vi "Host to DMA FIFO test.vi"() -> ()   [LabVIEW 2019]
uses:
  GlobalVars.vi
  <vilib>/FPGAPlugInAG/sbRIO-9606/niLvFpga_Open_sbRIO-9606.vi
  <vilib>/rvi/interface/common/dynamic/niFpgaDynamicAddResources.vi
  <vilib>/FPGAPlugInAG/Dynamic/niLvFpga_Abort_Dynamic.vi
  <vilib>/FPGAPlugInAG/Dynamic/niLvFpga_Reset_Dynamic.vi
  <vilib>/Utility/error.llb/Error Cluster From Error Code.vi
  <vilib>/rvi/errors/niLvFpgaAdjustHostInterfaceError.vi
  <vilib>/FPGAPlugInAG/Dynamic/niLvFpga_Run_Dynamic.vi
  <vilib>/FPGAPlugInAG/Dynamic/niLvFpga_Close_Dynamic.vi
  <vilib>/rvi/interface/nirviOpenFPGA/nirviOpenFPGA.xnode
  FPGA Bitfiles/sbriotest_MainFPGATarget_MainDMAFIFOtest_3lPTgoDMRHg.lvbitx
  Main DMA FIFO test.vi
  FPGA Bitfiles/sbriotest_SecondFPGATarget_AuxDMAFIFOtest_dfB-yokIQYE.lvbitx
  Aux DMA FIFO test.vi
  <vilib>/rvi/interface/nirviMethod/nirviMethod.xnode
  <vilib>/rvi/interface/nirviReadWriteControl/nirviReadWriteControl.xnode
  <vilib>/rvi/interface/nirviCloseFPGA/nirviCloseFPGA.xnode
  NiFpgaLv.dll
  <vilib>/rvi/interface/Simulation/niFpgaSimulationCallBeginRW.vi
  <vilib>/FPGAPlugInAG/Dynamic/niLvFpga_WriteFifo_Dynamic.vi
  <vilib>/rvi/errors/niLvFpgaMergeErrorWithErrorCode.vi
  <vilib>/FPGAPlugInAG/Dynamic/niLvFpga_ReadFifo_Dynamic.vi
panel:
  out "aux xt counter":u32
  out "both pass":bool
  out "GBIP total":i32
  out "xt counter":u32
  out "diff [us]":i32
  out "elapsed aux":u32
  out "GBIP command":string
  out "xt length":u32
  out "xt end":u32
  in  "stop":bool
  out "elapsed":u32
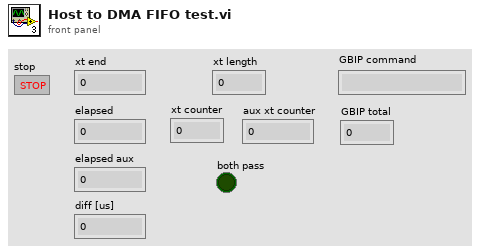
[diagram p1: front panel]
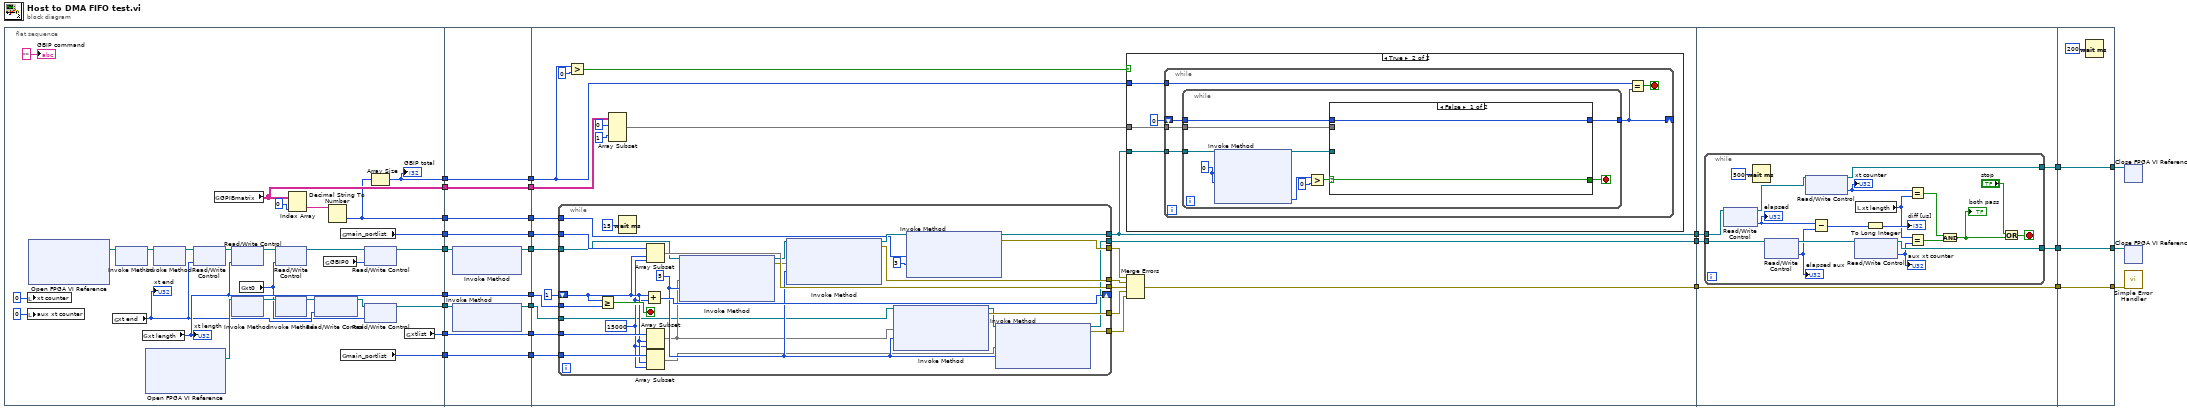
[diagram p0: block diagram]
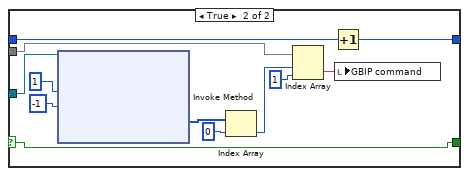
[diagram p3: hidden frame]
diagram:
  n1 = flat-sequence {
    tunnel: [w53] -> w21
    tunnel: [w52] -> w19
    tunnel: [w45] -> w17
    tunnel: [w49] -> w15
    tunnel: [w39] -> w13
    tunnel: [w36] -> w11
    tunnel: [w37] -> w9
    tunnel: [w32] -> w7
    tunnel: [w30] -> w6
    tunnel: w21 -> [w65]
    tunnel: [w65] -> w20
    tunnel: w19 -> [w64]
    tunnel: [w64] -> w18
    tunnel: w17 -> [w63]
    tunnel: [w63] -> w16
    tunnel: w15 -> [w62]
    tunnel: [w62] -> w14
    tunnel: w13 -> [w61]
    tunnel: [w61] -> w12
    tunnel: w11 -> [w60]
    tunnel: [w60] -> w10
    tunnel: w9 -> [w59]
    tunnel: [w59] -> w8
    tunnel: w7 -> [w58]
    tunnel: w6 -> [w57]
    tunnel: [w56] -> w5
    tunnel: [w55] -> w4
    tunnel: w20 -> [w88]
    tunnel: w18 -> [w87]
    tunnel: w16 -> [w84]
    tunnel: w14 -> [w70]
    tunnel: [w85] -> w25
    tunnel: w12 -> [w83]
    tunnel: [w77] -> w24
    tunnel: [w76] -> w22
    tunnel: w10 -> [w68]
    tunnel: w8 -> [w75]
    tunnel: w5 -> [w74]
    tunnel: w4 -> [w73]
    tunnel: w25 -> [w152]
    tunnel: w24 -> [w151]
    tunnel: w22 -> [w150]
    tunnel: [w154] -> w3
    tunnel: [w153] -> w2
    tunnel: [w151] -> w1
    tunnel: [w175] -> w23
    tunnel: [w176] -> w26
    tunnel: [w177] -> w27
    tunnel: w3 -> [w177]
    tunnel: w2 -> [w176]
    tunnel: w1 -> [w175]
    frame #0 {
      n2 = local write "xt counter"(u32 0 ("xt counter")) -> ()
      n3 = local write "aux xt counter"(u32 0 ("xt counter")) -> ()
      n4 = xnode "Open FPGA VI Reference"() -> ("FPGA VI Reference Out"=w54:refnum<k20>)  [unwired: 2 in, 1 out]
      n5 = global read "GlobalVars.vi" "xt end"() -> (w38:u32)
      "xt end" <- w38
      n6 = xnode "Invoke Method"("FPGA VI Reference In"=w54) -> ("FPGA VI Reference Out"=w40:refnum<k20>)  [unwired: 1 in, 1 out]
      n7 = global read "GlobalVars.vi" "xt length"() -> (w45:u32)
      "xt length" <- w45
      n8 = xnode "Open FPGA VI Reference"() -> ("FPGA VI Reference Out"=w48:refnum<k20>)  [unwired: 2 in, 1 out]
      n9 = xnode "Invoke Method"("FPGA VI Reference In"=w40) -> ("FPGA VI Reference Out"=w44:refnum<k20>)  [unwired: 1 in, 1 out]
      n10 = xnode "Read/Write Control"("FPGA VI Reference In"=w44, "xt end"=w38) -> ("FPGA VI Reference Out"=w46:refnum<k20>)  [unwired: 1 in, 1 out]
      n11 = global read "GlobalVars.vi" "GPIBmatrix"() -> (w49:string[][])
      n12 = xnode "Read/Write Control"("FPGA VI Reference In"=w46, "xt total"=w45) -> ("FPGA VI Reference Out"=w35:refnum<k20>)  [unwired: 1 in, 1 out]
      n13 = xnode "Invoke Method"("FPGA VI Reference In"=w48) -> ("FPGA VI Reference Out"=w41:refnum<k20>)  [unwired: 1 in, 1 out]
      n14 = global read "GlobalVars.vi" "xt0"() -> (w29:u32)
      n15 = xnode "Read/Write Control"("FPGA VI Reference In"=w35, "xt0"=w29) -> ("FPGA VI Reference Out"=w33:refnum<k20>)  [unwired: 1 in, 1 out]
      n16 = xnode "Invoke Method"("FPGA VI Reference In"=w41) -> ("FPGA VI Reference Out"=w43:refnum<k20>)  [unwired: 1 in, 1 out]
      n17 = Index Array(array=w49, index (col)=0 ("disabled index (col)")) -> (element=w50:string[])  [unwired: 1 in]
      n18 = xnode "Read/Write Control"("FPGA VI Reference In"=w43, "xt end aux"=w38) -> ("FPGA VI Reference Out"=w34:refnum<k20>)  [unwired: 1 in, 1 out]
      n19 = global read "GlobalVars.vi" "GBIP0"() -> (w31:u32)
      n20 = Decimal String To Number(string=w50) -> (number=w37:i32[])  [unwired: 2 in, 1 out]
      n21 = global read "GlobalVars.vi" "main_portlist"() -> (w52:u32[])
      n22 = global read "GlobalVars.vi" "main_portlist"() -> (w39:u32[])
      n23 = xnode "Read/Write Control"("FPGA VI Reference In"=w33, "GPIB0"=w31) -> ("FPGA VI Reference Out"=w32:refnum<k20>)  [unwired: 1 in, 1 out]
      n24 = xnode "Read/Write Control"("FPGA VI Reference In"=w34, "xt0"=w29) -> ("FPGA VI Reference Out"=w30:refnum<k20>)  [unwired: 1 in, 1 out]
      n25 = Array Size(array=w37) -> (size(s)=w36:i32)
      "GBIP total" <- w36
      n26 = global read "GlobalVars.vi" "xtlist"() -> (w53:u32[])
      "GBIP command" <- "" ("GBIP command")
    }
    frame #1 {
      n27 = xnode "Invoke Method"("FPGA VI Reference In"=w58) -> ("FPGA VI Reference Out"=w56:refnum<k20>)  [unwired: 2 in, 1 out]
      n28 = xnode "Invoke Method"("FPGA VI Reference In"=w57) -> ("FPGA VI Reference Out"=w55:refnum<k20>)  [unwired: 2 in, 1 out]
    }
    frame #2 {
      n29 = while {
        tunnel: [w149] -> w81
        tunnel: [w148] -> w80
        tunnel: w88 -> [w146]
        tunnel: w87 -> [w147]
        shift-right: [w145] -> _
        shift-left: 1 -> [w127]
        tunnel: w84 -> [w144]
        tunnel: [w142] -> w82
        tunnel: [w138] -> w79
        tunnel: [w137] -> w78
        tunnel: [w132] -> w85
        tunnel: [w131] -> w76
        tunnel: w83 -> [w130]
        tunnel: w75 -> [w128]
        tunnel: w74 -> [w124]
        tunnel: w73 -> [w123]
        stop <- w143 stop-if-true
        w126 = 15000
        w140 = 5
        n30 = Greater Or Equal?(x=w127, y=w144) -> (x >= y?=w143:bool)
        n31 = Wait (ms)(milliseconds to wait=u32 15) -> ()  [unwired: 1 out]
        n32 = Add(x=w127, y=w126) -> (x+y=w145:i32)
        n33 = Array Subset(array=w147, index=w127, length=w126) -> (w139:u32[])
        n34 = Array Subset(array=w146, index=w127, length=w126) -> (w125:u32[])
        n35 = Array Subset(array=w130, index=w127, length=w126) -> (w129:u32[])
        n36 = xnode "Invoke Method"("FPGA VI Reference In"=w124, "Data"=w125, "Timeout (ms)"=w140) -> ("FPGA VI Reference Out"=w135:refnum<k20>, "error out"=w148:errorcluster)  [unwired: 1 in, 1 out]
        n37 = xnode "Invoke Method"("FPGA VI Reference In"=w135, "Data"=w139, "Timeout (ms)"=w140) -> ("FPGA VI Reference Out"=w134:refnum<k20>, "error out"=w149:errorcluster)  [unwired: 1 in, 1 out]
        n38 = xnode "Invoke Method"("FPGA VI Reference In"=w123, "Data"=w125, "Timeout (ms)"=w140) -> ("FPGA VI Reference Out"=w133:refnum<k20>, "error out"=w138:errorcluster)  [unwired: 1 in, 1 out]
        n39 = xnode "Invoke Method"("FPGA VI Reference In"=w134, "Data"=w128, "Timeout (ms)"=3) -> ("FPGA VI Reference Out"=w131:refnum<k20>, "error out"=w142:errorcluster)  [unwired: 1 in, 1 out]
        n40 = xnode "Invoke Method"("FPGA VI Reference In"=w133, "Data"=w129, "Timeout (ms)"=w140) -> ("FPGA VI Reference Out"=w132:refnum<k20>, "error out"=w137:errorcluster)  [unwired: 1 in, 1 out]
      }
      n41 = Greater?(x=w68, y=0) -> (0:w66:bool)
      n42 = Array Subset(array=w70, index (row)=0 ("index"), index (col)=1 ("index")) -> (w69:string[][])  [unwired: 2 in]
      n43 = case shown="True" w66 {
        tunnel: w76 -> [_ w92]
        tunnel: w69 -> [_ w91]
        tunnel: w68 -> [_ w90]
        frame False {
        }
        frame True {
          n44 = while {
            tunnel: w92 -> [w98]
            tunnel: w91 -> [w97]
            shift-right: [w94] -> _
            shift-left: 0 -> [w96]
            tunnel: w90 -> [w93]
            stop <- w95 stop-if-true
            n45 = while {
              tunnel: w98 -> [w108]
              tunnel: w97 -> [w107]
              tunnel: w96 -> [w102]
              tunnel: [w101] -> w94
              stop <- w100 stop-if-true
              w99 = 0 ("Timeout (ms)")
              n46 = xnode "Invoke Method"("FPGA VI Reference In"=w108, "Number of Elements"=w99, "Timeout (ms)"=w99) -> ("FPGA VI Reference Out"=w106:refnum<k20>, "Elements Remaining"=w104:u32)  [unwired: 1 in, 2 out]
              n47 = Greater?(x=w104, y=u16 0) -> (0:w103:bool)
              n48 = case shown="False" w103 {
                selector: w103 -> [w109 w111]
                tunnel: w107 -> [_ w122]
                tunnel: w106 -> [_ w121]
                tunnel: w102 -> [w110 w113]
                tunnel: [w110 w112] -> w101
                tunnel: [w109 w111] -> w100
                frame False {
                }
                frame True {
                  n49 = xnode "Invoke Method"("FPGA VI Reference In"=w121, "Number of Elements"=u32 1, "Timeout (ms)"=-1) -> ("Data"=w118:u16[])  [unwired: 1 in, 3 out]
                  n50 = Index Array(array=w118, index=0) -> (element=w116:u16)
                  n51 = Index Array(array=w122, index (row)=w116, index (col)=1 ("disabled index (col)")) -> (element=w114:string)
                  n52 = Increment(x=w113) -> (x+1=w112:i32)
                  n53 = local write "GBIP command"(w114) -> ()
                }
              }
            }
            n54 = Equal?(x=w93, y=w94) -> (x = y?=w95:bool)
          }
        }
      }
      n55 = Merge Errors(w82, w81, w80, w79, w78) -> (w77:errorcluster)
    }
    frame #3 {
      n56 = while {
        tunnel: [w163] -> w154
        tunnel: [w167] -> w153
        tunnel: w152 -> [w166]
        tunnel: w150 -> [w164]
        stop <- w161 stop-if-true
        n57 = xnode "Read/Write Control"("FPGA VI Reference In"=w164) -> ("FPGA VI Reference Out"=w168:refnum<k20>, "elapsed"=w165:u32)  [unwired: 1 in, 1 out]
        "elapsed" <- w165
        n58 = Wait (ms)(milliseconds to wait=u32 500) -> ()  [unwired: 1 out]
        n59 = xnode "Read/Write Control"("FPGA VI Reference In"=w166) -> ("FPGA VI Reference Out"=w173:refnum<k20>, "elapsed"=w172:u32)  [unwired: 1 in, 1 out]
        "elapsed aux" <- w172
        n60 = xnode "Read/Write Control"("FPGA VI Reference In"=w168) -> ("FPGA VI Reference Out"=w167:refnum<k20>, "xt counter"=w159:u32)  [unwired: 1 in, 1 out]
        "xt counter" <- w159
        n61 = Subtract(x=w165, y=w172) -> (x-y=w171:u32)
        n62 = xnode "Read/Write Control"("FPGA VI Reference In"=w173) -> ("FPGA VI Reference Out"=w163:refnum<k20>, "xt counter"=w160:u32)  [unwired: 1 in, 1 out]
        "aux xt counter" <- w160
        n63 = local read "xt length"() -> (w158:u32)
        n64 = To Long Integer(number=w171) -> (32bit integer=→"diff [us]":i32)
        n65 = Equal?(x=w159, y=w158) -> (x = y?=w157:bool)
        n66 = Equal?(x=w158, y=w160) -> (x = y?=w156:bool)
        n67 = And(x=w157, y=w156) -> (x .and. y?=w155:bool)
        "both pass" <- w155
        n68 = Or(x="stop", y=w155) -> (x .or. y?=w161:bool)
      }
    }
    frame #4 {
      n69 = Wait (ms)(milliseconds to wait=u32 200) -> ()  [unwired: 1 out]
    }
  }
  n70 = xnode "Close FPGA VI Reference"("FPGA VI Reference In"=w26) -> ()  [unwired: 1 in, 1 out]
  n71 = xnode "Close FPGA VI Reference"("FPGA VI Reference In"=w27) -> ()  [unwired: 1 in, 1 out]
  n72 = call <vilib>:"Simple Error Handler.vi"("error in (no error)"=w23) -> ()  [unwired: 4 in, 5 out]
